vi "Update Filtered Message Log MHLC.vi"(8 "error in (no error)":errorcluster, 11 "Message Log in":refnum<class "Message Log.lvclass">) -> (0 "error out":errorcluster, 3 "Message Log out":refnum<class "Message Log.lvclass">)   [LabVIEW 2017, in "Message Log.lvclass"]
doc: "Filter the UI Message Log and update the UI Message Log with filtered data"
uses:
  Message Log.lvclass
  Message Log.lvclass/Message Log.ctl
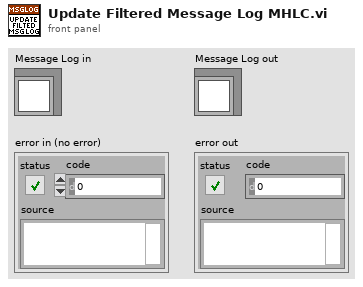
[diagram p1: front panel]
types:
  T1 = typedef "Message Log.lvclass/Message Log Filter Data.ctl" = cluster{"Element":string, "Column":T2, "Filter Type":T3}
  T2 = typedef "Message Log.lvclass/Message Log Columns.ctl" = enum16{"Count (sec)", "Time/Date", "Enque Worker", "Enque Case", "Deque Worker", "Deque Case", "Priority", "Message"}
  T3 = typedef "Message Log.lvclass/String Filter Type.ctl" = enum16{"string only", "match pattern"}
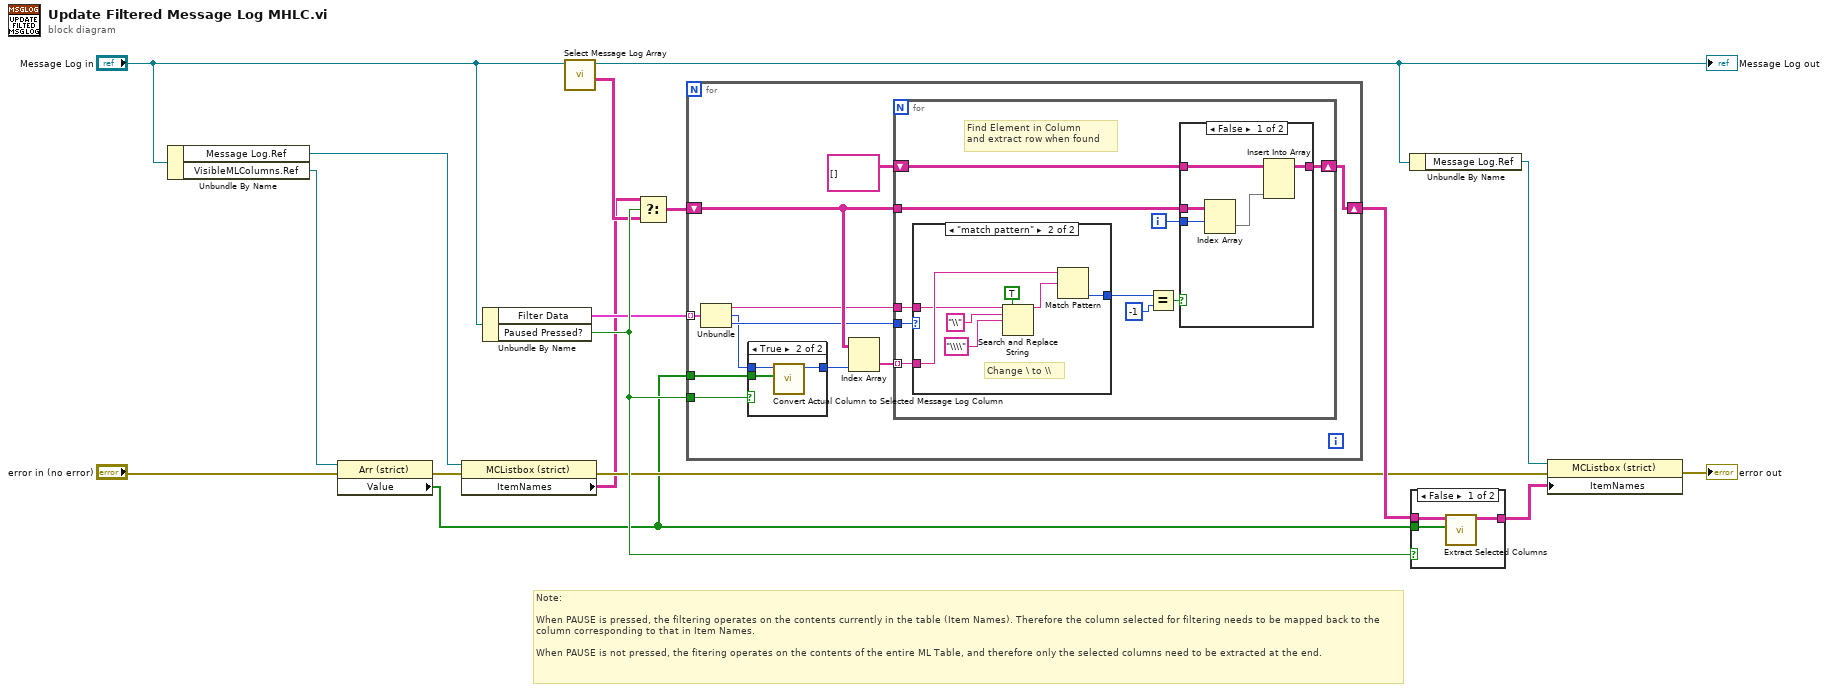
[diagram p0: block diagram]
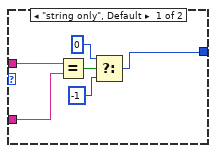
[diagram p4: hidden frame]
diagram:
  # "Note:\n\nWhen PAUSE is pressed, the filtering operates on the contents currently in the table (Item Names). Therefore the column selected for filtering needs to be mapped back to the column corresponding to that in Item Names.\n\nWhen PAUSE is not pressed, the fitering operates on the contents of the entire ML Table, and therefore only the selected columns need to be extracted at the end."
  n1 = Unbundle By Name("Message Log in") -> ("Message Log.Ref"=w4:refnum<vi>, "VisibleMLColumns.Ref"=w2:refnum<vi>)
  n2 = property class="Arr (strict)"(reference=w2, error in="error in (no error)") -> (error out=w3:errorcluster, "Value"=w1:bool[])  [unwired: 1 out]
  n3 = property class="MCListbox (strict)"(reference=w4, error in=w3) -> (error out=w6:errorcluster, "ItemNames"=w5:string[][])  [unwired: 1 out]
  n4 = Unbundle By Name("Message Log in") -> ("Filter Data"=w14:T1[], "Paused Pressed?"=w17:bool)
  n5 = call "Select Message Log Array.vi"("Message Log in"="Message Log in") -> ("Selected Array"=w15:string[][], "Message Log out"=w12:refnum<class "Message Log.lvclass">)  [unwired: 9 in]
  "Message Log out" <- w12
  n6 = Select(t=w5, s=w17, f=w15) -> (s? t:f=w13:string[][])
  n7 = for {
    tunnel: w14 -> [w24] mode=indexing
    shift-right: [w26] -> w16
    shift-left: w13 -> [w25]
    tunnel: w1 -> [w21]
    tunnel: w17 -> [w18]
    n8 = Unbundle(w24) -> ("Element"=w23:string, "Column"=w20:T2, "Filter Type"=w22:T3)
    n9 = case shown="True" w18 {
      tunnel: w21 -> [_ w32]
      tunnel: w20 -> [w29 w31]
      tunnel: [w29 w30] -> w19
      frame False {
      }
      frame True {
        n10 = call "Convert Actual Column to Selected Message Log Column.vi"("Visible ML Columns"=w32, "Actual Column"=w31) -> ("Selected Column"=w30:i32)  [unwired: 9 in]
      }
    }
    n11 = Index Array(array=w25, index (col)=w19) -> (element=w28:string[])  [unwired: 1 in]
    n12 = for {
      tunnel: w23 -> [w34]
      tunnel: w28 -> [w35] mode=indexing
      tunnel: w25 -> [w41]
      shift-right: [w39] -> w26
      shift-left: string[][] [] ("Sorted Array Out") -> [w42]
      tunnel: w22 -> [w33]
      i -> [w40]
      # "Find Element in Column\nand extract row when found"
      n13 = case shown="\"match pattern\"" w33 {
        tunnel: [w46 w55] -> w37
        tunnel: w35 -> [w47 w51]
        tunnel: w34 -> [w48 w50]
        frame "string only", Default {
          n14 = Equal?(x=w48, y=w47) -> (x = y?=w45:bool)
          n15 = Select(t=0 ("y"), s=w45, f=-1 ("y")) -> (s? t:f=w46:i32)
        }
        frame "match pattern" {
          # "Change \\ to \\\\"
          n16 = Search and Replace String(replace all?=TRUE ("replace all? (F)"), input string=w50, search string="\\", replace string="\\\\" ("replace string (\"\")")) -> (result string=w49:string)  [unwired: 4 in, 3 out]
          n17 = Match Pattern(string=w51, regular expression=w49) -> (offset past match=w55:i32)  [unwired: 1 in, 3 out]
        }
      }
      n18 = Equal?(x=w37, y=-1) -> (x = y?=w38:bool)
      n19 = case shown="False" w38 {
        tunnel: w42 -> [w60 w61]
        tunnel: w41 -> [w59 _]
        tunnel: w40 -> [w58 _]
        tunnel: [w56 w61] -> w39
        frame False {
          n20 = Index Array(array=w59, index (row)=w58) -> (element=w57:string[])  [unwired: 1 in]
          n21 = Insert Into Array(array=w60, new element=w57) -> (w56:string[][])  [unwired: 2 in]
        }
        frame True {
        }
      }
    }
  }
  n22 = Unbundle By Name(w12) -> ("Message Log.Ref"=w11:refnum<vi>)
  n23 = case shown="False" w17 {
    tunnel: [w64 w65] -> w10
    tunnel: w16 -> [w63 w65]
    tunnel: w1 -> [w62 _]
    frame False {
      n24 = call "Extract Selected Columns.vi"("Visible ML Columns"=w62, "Array in"=w63) -> ("Selected Columns out"=w64:string[][])  [unwired: 9 in]
    }
    frame True {
    }
  }
  n25 = property class="MCListbox (strict)"(reference=w11, error in=w6, "ItemNames"=w10) -> (error out=→"error out":errorcluster)  [unwired: 1 out]
